vi "DAQ.showUI.vi"(8 "error in (no error)":errorcluster, 10 "show UI?":T1, 11 "Instrument.DAQ":refnum<class "Instrument.DAQ.lvclass">) -> (0 "error out":errorcluster, 3 "Instrument.DAQ out":refnum<class "Instrument.DAQ.lvclass">)   [LabVIEW 2019, in "Instrument.Lockin.lvlib" / "Instrument.DAQ.lvclass"]
doc: "---------------------------------------------------------------\nJKI State Machine Objects™\nhttp://jki.net/state-machine-objects/\nCopyright (C) 2005-2015, JKI <info@jki.net>\nALL RIGHTS RESERVEDJKI State Machine Objects (SMO) 1.0.0.4\nJKI - JKI\nCopyright (c) 2015, JKI"
uses:
  Instrument.DAQ.lvclass
  Typedefs/PrivateEvents--DAQ.showUI.ctl
  Instrument.DAQ.lvclass/Instrument.DAQ.ctl
panel:
  # "For instructions on how to use the JKI State Machine Objects, examples and video tutorials, visit:\nhttp://jki.net/state-machine-objects/\n\nJKI State Machine Objects™\nhttp://jki.net/state-machine-objects/\nCopyright (C) 2005-2015, JKI <info@jki.net>\nALL RIGHTS RESERVED"
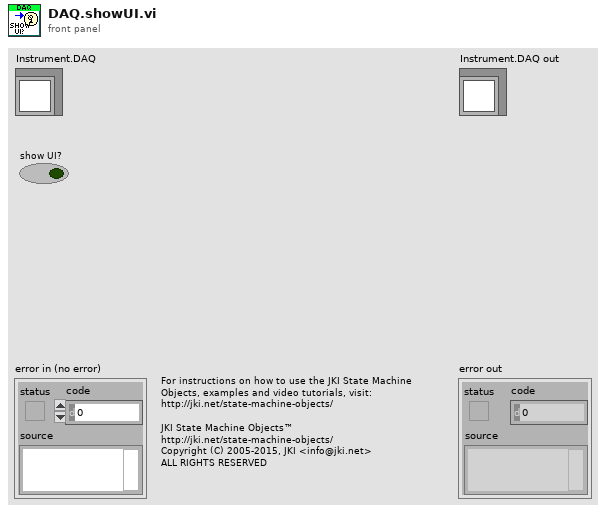
[diagram p1: front panel]
types:
  T1 = typedef "Instrument.Lockin.lvlib/Instrument.DAQ.lvclass/PrivateEvents--DAQ.showUI.ctl" = bool
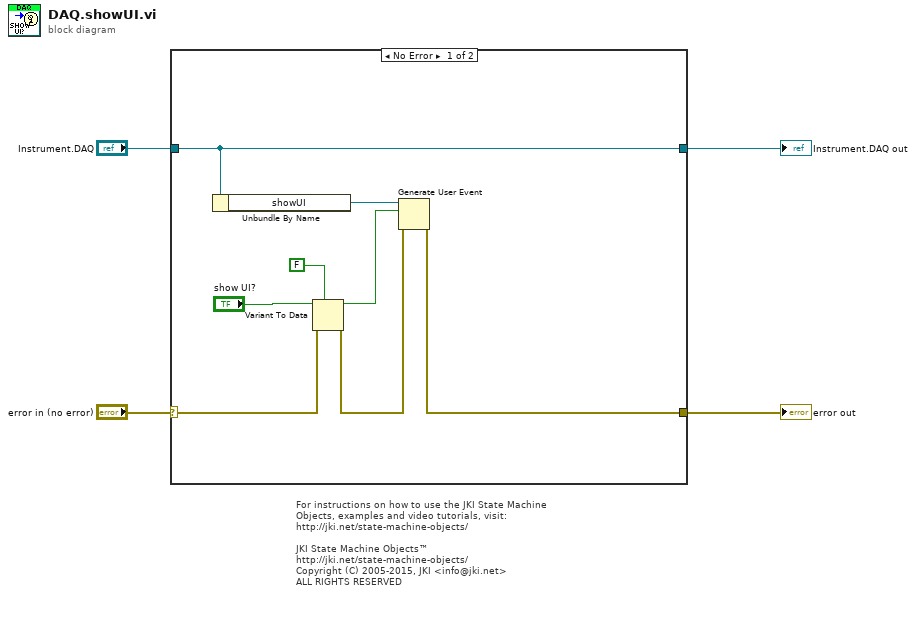
[diagram p0: block diagram]
diagram:
  # "For instructions on how to use the JKI State Machine Objects, examples and video tutorials, visit:\nhttp://jki.net/state-machine-objects/\n\nJKI State Machine Objects™\nhttp://jki.net/state-machine-objects/\nCopyright (C) 2005-2015, JKI <info@jki.net>\nALL RIGHTS RESERVED"
  n1 = case shown="No Error" "error in (no error)" {
    selector: "error in (no error)" -> [w6 w14]
    tunnel: [w11 w14] -> w3
    tunnel: [w10 w13] -> w4
    tunnel: "Instrument.DAQ" -> [w10 w13]
    frame No Error {
      n2 = Unbundle By Name(w10) -> ("showUI"=w12:refnum<user-event>)
      n3 = Variant To Data(error in=w6, type=T1 FALSE ("showDAQUI"), Variant="show UI?") -> (data=w7:T1, error out=w5:errorcluster)
      n4 = Generate User Event(user event=w12, event data cluster=w7, error in=w5) -> (error out=w11:errorcluster)  [unwired: 1 in, 1 out]
    }
    frame Error {
    }
  }
  "error out" <- w3
  "Instrument.DAQ out" <- w4
